vi "Post-Install Library Setup.vi"(10 "Variant":variant) -> (0 "error out":errorcluster)   [LabVIEW 2013]
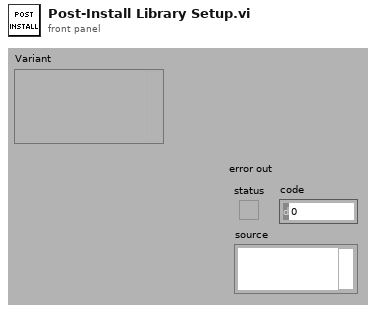
[diagram p1: front panel]
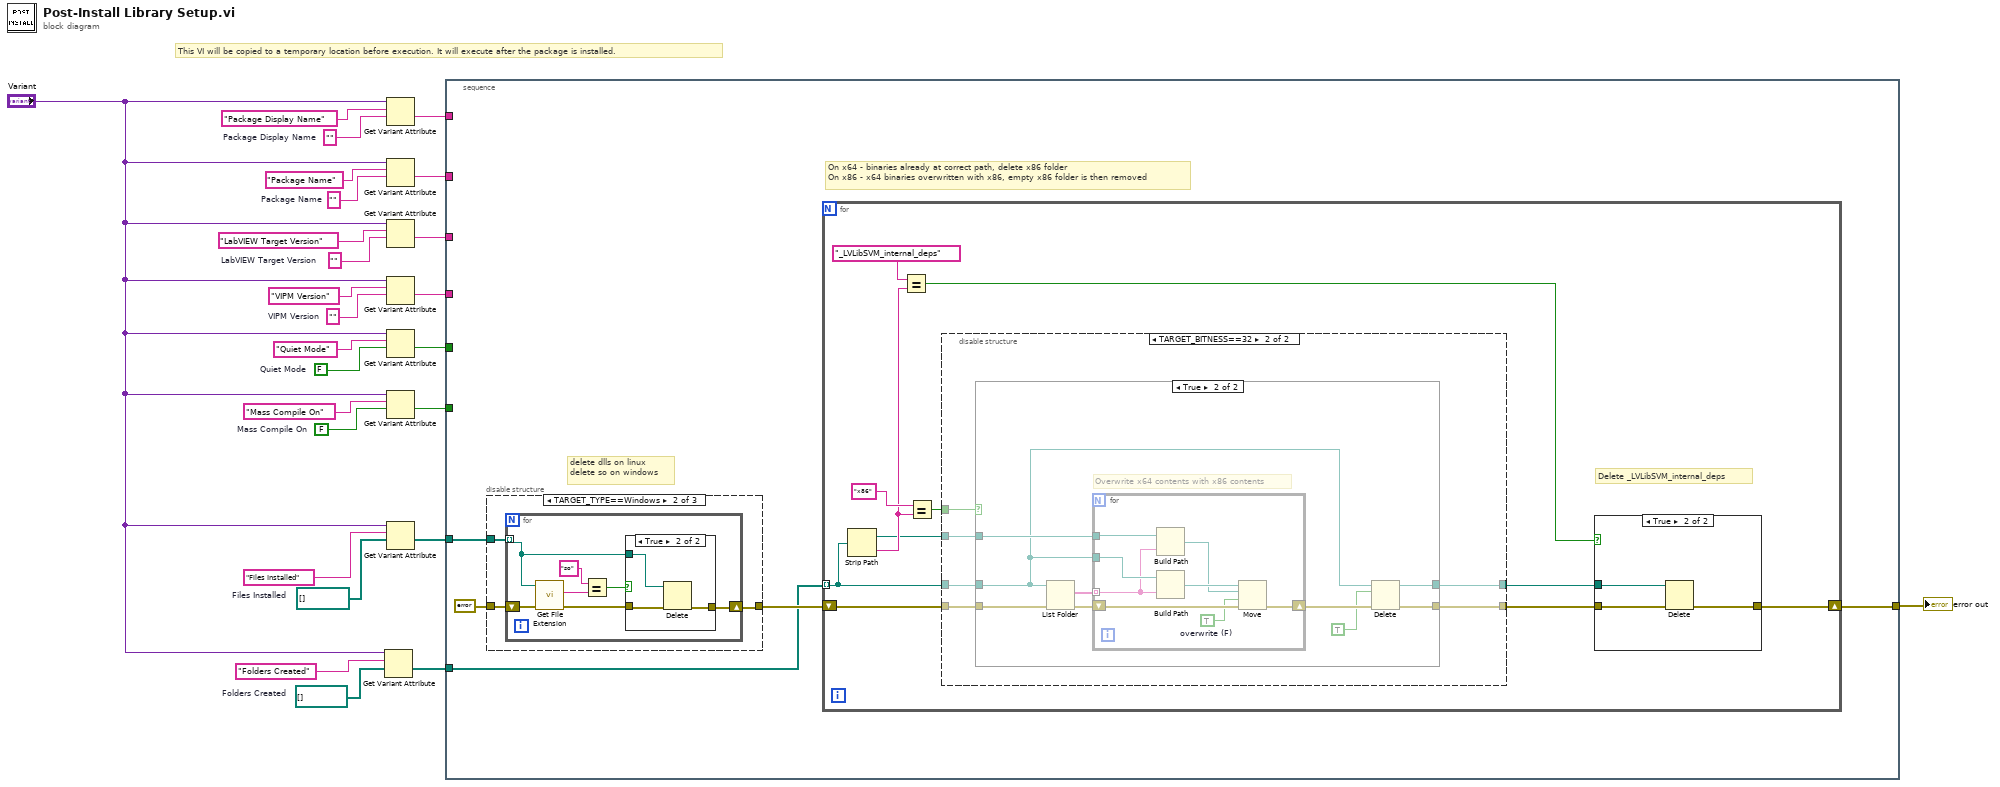
[diagram p0: block diagram]
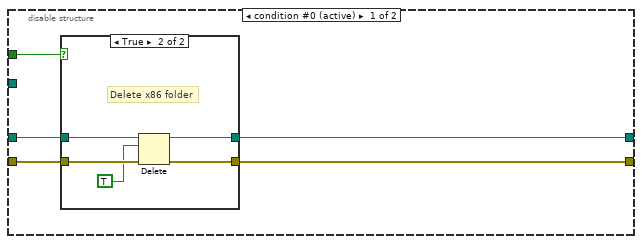
[diagram p3: hidden frame]
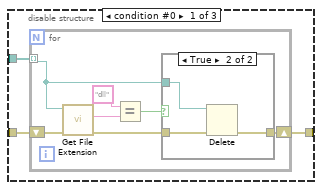
[diagram p6: hidden frame]
diagram:
  w2 = path[] []  # Folders Created
  w3 = path[] []  # Files Installed
  w9 = FALSE  # Mass Compile On
  w10 = ""  # Package Display Name
  w17 = FALSE  # Quiet Mode
  w20 = ""  # VIPM Version
  w22 = ""  # LabVIEW Target Version
  w24 = ""  # Package Name
  # "This VI will be copied to a temporary location before execution. It will execute after the package is installed."
  n1 = Get Variant Attribute(Variant="Variant", name="Folders Created", default value (empty Variant)=w2) -> (value=w7:path[])  [unwired: 1 in, 3 out]
  n2 = Get Variant Attribute(Variant="Variant", name="Package Display Name", default value (empty Variant)=w10) -> (value=w16:string)  [unwired: 1 in, 3 out]
  n3 = Get Variant Attribute(Variant="Variant", name="Package Name", default value (empty Variant)=w24) -> (value=w15:string)  [unwired: 1 in, 3 out]
  n4 = Get Variant Attribute(Variant="Variant", name="LabVIEW Target Version", default value (empty Variant)=w22) -> (value=w14:string)  [unwired: 1 in, 3 out]
  n5 = Get Variant Attribute(Variant="Variant", name="VIPM Version", default value (empty Variant)=w20) -> (value=w13:string)  [unwired: 1 in, 3 out]
  n6 = Get Variant Attribute(Variant="Variant", name="Quiet Mode", default value (empty Variant)=w17) -> (value=w12:bool)  [unwired: 1 in, 3 out]
  n7 = Get Variant Attribute(Variant="Variant", name="Mass Compile On", default value (empty Variant)=w9) -> (value=w11:bool)  [unwired: 1 in, 3 out]
  n8 = Get Variant Attribute(Variant="Variant", name="Files Installed", default value (empty Variant)=w3) -> (value=w6:path[])  [unwired: 1 in, 3 out]
  n9 = stacked-sequence {
    tunnel: w16 -> [_]
    tunnel: w15 -> [_]
    tunnel: w14 -> [_]
    tunnel: w13 -> [_]
    tunnel: w12 -> [_]
    tunnel: w11 -> [_]
    tunnel: w6 -> [w30]
    tunnel: w7 -> [w28]
    tunnel: [w27] -> w1
    frame #0 {
      # "On x64 - binaries already at correct path, delete x86 folder\nOn x86 - x64 binaries overwritten with x86, empty x86 folder is then removed"
      # "delete dlls on linux\ndelete so on windows"
      n10 = disable-structure shown="TARGET_TYPE==Windows" {
        disable-tunnel: errorcluster {"status"=FALSE, "code"=0, "source"=""} ("error out") -> [w86 w100 w112]
        disable-tunnel: w30 -> [w85 w99 _]
        disable-tunnel: [w84 w98 w112] -> w29
        frame condition #0 {
          n11 = for {
            tunnel: w85 -> [w87] mode=indexing
            shift-right: [w88] -> w84
            shift-left: w86 -> [w93]
            n12 = call <vilib>:"Get File Extension.vi"("error in (no error)"=w93, "file"=w87) -> ("error out"=w92:errorcluster, "lowercase file extension"=w91:string)  [unwired: 6 in, 2 out]
            n13 = Equal?(x="dll", y=w91) -> (x = y?=w90:bool)
            n14 = case shown="True" w90 {
              tunnel: w92 -> [w94 w97]
              tunnel: [w94 w96] -> w88
              tunnel: w87 -> [_ w95]
              frame False {
              }
              frame True {
                n15 = Delete(path (use dialog)=w95, error in=w97) -> (error out=w96:errorcluster)  [unwired: 3 in, 2 out]
              }
            }
          }
        }
        frame condition #1 (active) {
          n16 = for {
            tunnel: w99 -> [w101] mode=indexing
            shift-right: [w102] -> w98
            shift-left: w100 -> [w107]
            n17 = call <vilib>:"Get File Extension.vi"("error in (no error)"=w107, "file"=w101) -> ("error out"=w106:errorcluster, "lowercase file extension"=w105:string)  [unwired: 6 in, 2 out]
            n18 = Equal?(x="so", y=w105) -> (x = y?=w104:bool)
            n19 = case shown="True" w104 {
              tunnel: w106 -> [w108 w111]
              tunnel: [w108 w110] -> w102
              tunnel: w101 -> [_ w109]
              frame False {
              }
              frame True {
                n20 = Delete(path (use dialog)=w109, error in=w111) -> (error out=w110:errorcluster)  [unwired: 3 in, 2 out]
              }
            }
          }
        }
        frame condition #2 {
        }
      }
      n21 = for {
        shift-right: [w35] -> w27
        shift-left: w29 -> [w40]
        tunnel: w28 -> [w39] mode=indexing
        # "Delete _LVLibSVM_internal_deps"
        n22 = Strip Path(path=w39) -> (stripped path=w32:path, name=w38:string)
        n23 = Equal?(x="_LVLibSVM_internal_deps" ("name or relative path"), y=w38) -> (x = y?=w34:bool)
        n24 = Equal?(x="x86", y=w38) -> (x = y?=w42:bool)
        n25 = disable-structure shown="TARGET_BITNESS==32" {
          disable-tunnel: w42 -> [w51 w64]
          disable-tunnel: w40 -> [w50 w63]
          disable-tunnel: w39 -> [w49 w62]
          disable-tunnel: [w48 w59] -> w33
          disable-tunnel: [w47 w60] -> w36
          disable-tunnel: w32 -> [_ w61]
          frame condition #0 (active) {
            n26 = case shown="True" w51 {
              tunnel: w50 -> [w52 w58]
              tunnel: w49 -> [w53 w57]
              tunnel: [w52 w56] -> w47
              tunnel: [w53 w55] -> w48
              frame False {
              }
              frame True {
                # "Delete x86 folder"
                n27 = Delete(path (use dialog)=w57, entire hierarchy (F)=TRUE, error in=w58) -> (deleted path=w55:path, error out=w56:errorcluster)  [unwired: 2 in, 1 out]
              }
            }
          }
          frame condition #1 {
            n28 = case shown="True" w64 {
              tunnel: w63 -> [w66 w75]
              tunnel: w62 -> [w65 w69]
              tunnel: w61 -> [_ w72]
              tunnel: [w66 w70] -> w60
              tunnel: [w65 w67] -> w59
              frame False {
              }
              frame True {
                # "Overwrite x64 contents with x86 contents"
                n29 = List Folder(path=w69, error in=w75) -> (filenames=w73:string[], error out=w74:errorcluster)  [unwired: 2 in, 2 out]
                n30 = for {
                  tunnel: w73 -> [w79] mode=indexing
                  tunnel: w69 -> [w83]
                  tunnel: w72 -> [w80]
                  shift-right: [w76] -> w71
                  shift-left: w74 -> [w82]
                  w77 = TRUE  # overwrite (F)
                  n31 = Build Path(base path=w80, name or relative path=w79) -> (appended path=w78:path)
                  n32 = Build Path(base path=w83, name or relative path=w79) -> (appended path=w81:path)
                  n33 = Move(source path=w81, error in=w82, 9:w77, 10:w78) -> (error out=w76:errorcluster)  [unwired: 1 in, 2 out]
                }
                n34 = Delete(path (use dialog)=w69, entire hierarchy (F)=TRUE, error in=w71) -> (deleted path=w67:path, error out=w70:errorcluster)  [unwired: 2 in, 1 out]
              }
            }
          }
        }
        n35 = case shown="True" w34 {
          tunnel: w36 -> [w43 w46]
          tunnel: [w43 w45] -> w35
          tunnel: w33 -> [_ w44]
          frame False {
          }
          frame True {
            n36 = Delete(path (use dialog)=w44, error in=w46) -> (error out=w45:errorcluster)  [unwired: 3 in, 2 out]
          }
        }
      }
    }
  }
  "error out" <- w1
